vi "Create.vi"(8 "error in (no error)":errorcluster, 9 "Control Values":cluster{"Name":string, "Control Data":variant}[](array[cluster]), 10 "VI Name":string) -> (0 "error out":errorcluster, 3 "Parametric VI Call Out":refnum<class "Parametric VI Call.lvclass">)   [LabVIEW 2020, in "Parametric VI Call.lvclass"]
uses:
  Parametric VI Call.lvclass
  Parametric VI Call.lvclass/Parametric VI Call.ctl
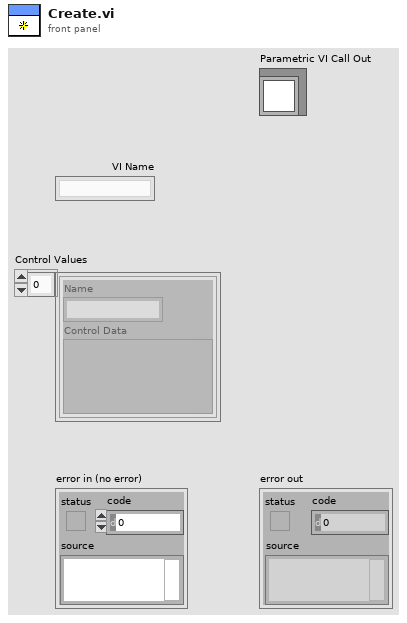
[diagram p1: front panel]
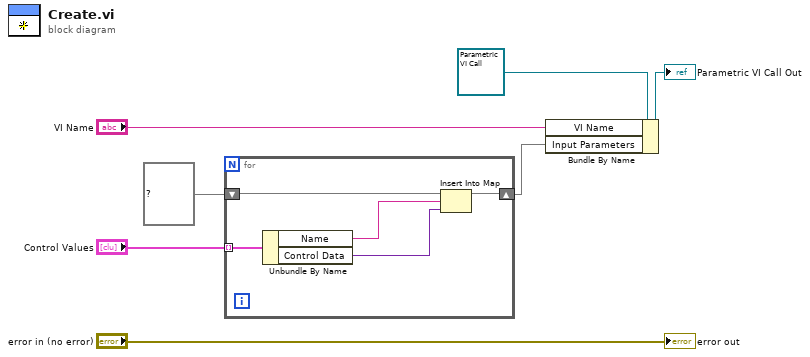
[diagram p0: block diagram]
diagram:
  n1 = for {
    shift-right: [w11] -> w1
    shift-left: map{string, variant} {} ("map") -> [w12]
    tunnel: "Control Values" -> [w10] mode=indexing
    n2 = Unbundle By Name(w10) -> ("Name"=w9:string, "Control Data"=w8:variant)
    n3 = Insert Into Map(map in=w12, key=w9, value=w8) -> (map out=w11:map{string, variant})  [unwired: 2 out]
  }
  n4 = Bundle By Name(cluster=refnum<class "Parametric VI Call.lvclass"> refnum ("Parametric VI Call"), "VI Name"="VI Name", "Input Parameters"=w1) -> (→"Parametric VI Call Out":refnum<class "Parametric VI Call.lvclass">)
  "error out" <- "error in (no error)"
